vi "VITester_Item_OnCommand.vi"(10 "Command ID":string, 11 "Object":T1) -> ()   [LabVIEW 2009]
uses:
  Support/VITester Project Item Ref.ctl
panel:
  out "error out":errorcluster
  in  "error in":errorcluster
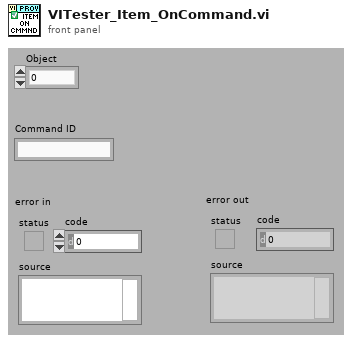
[diagram p1: front panel]
types:
  T1 = typedef "VITester Project Item Ref.ctl" = u64
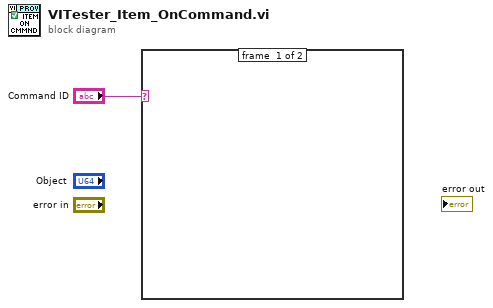
[diagram p0: block diagram]
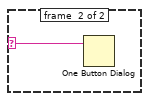
[diagram p2: hidden frame]
diagram:
  n1 = case shown="\"MY_SECONDARY_POPUP\"" "Command ID" {
    selector: "Command ID" -> [_ w2]
    frame #0 {
    }
    frame #1 {
      n2 = One Button Dialog(message=w2) -> ()  [unwired: 1 in, 1 out]
    }
  }
